vi "FF Target IN POLARIS Vision.vi"() -> ()   [LabVIEW 2009]
uses:
  IMAQdx Cam/IMAQdx Cam.lvclass
  XDisplay/POLARIS IMAQ Display.xctl
  XDisplay/Properties/ImageSource.ctl
  Utility/POLARIS Vision utility.lvlib
  Analyze Classes/Analyze Timer/Analyze Timer.lvclass
panel:
  in  "Amplifier":enum16{"CW", "A2", "A2 1.6x", "A3", "A4", "A5"}(ring)=enum."A4"
  out "error load settings":errorcluster
  in  "stop2":bool
  in  "Config Dir":path
  in  "Prefix":string
  in  "WorkDir":path
  out "XDisplay":cluster{"Image":T1}(xcontrol)
  in  "stop":bool
  in  "Camera Name":string
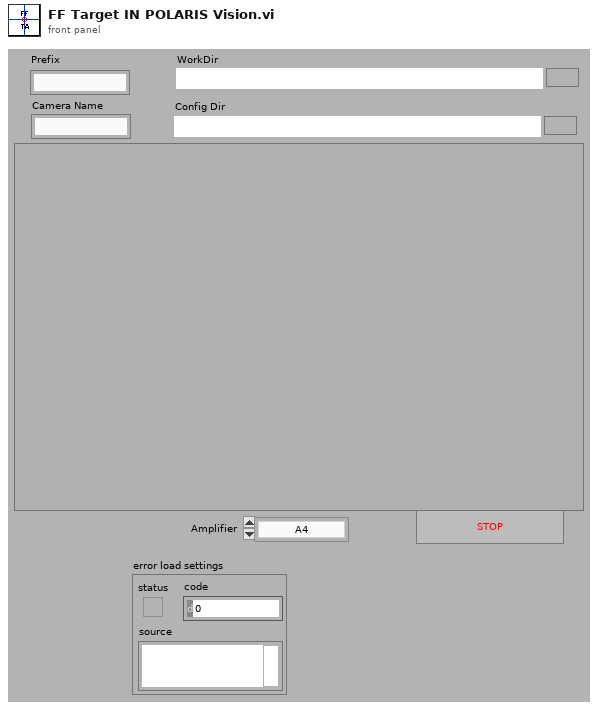
[diagram p1: front panel]
types:
  T1 = typedef "IMAQ Image.ctl" = refnum<image>
  T2 = typedef "POLARIS IMAQ Display.xctl/ImageSource.ctl" = enum16{"Camera", "File"}
  T3 = typedef "Image Type" = u32
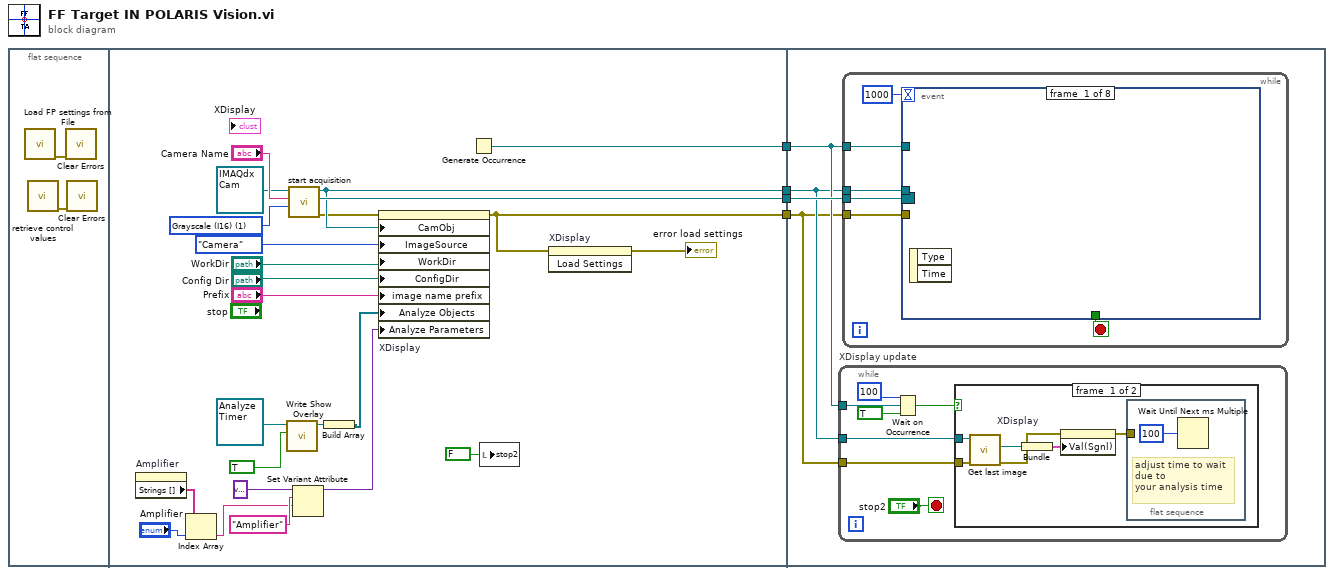
[diagram p0: block diagram]
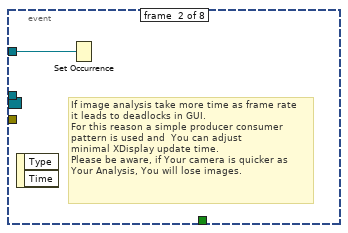
[diagram p3: hidden frame]
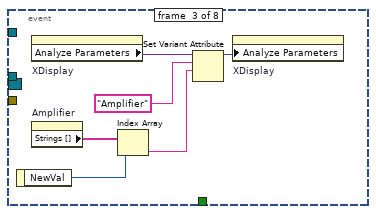
[diagram p4: hidden frame]
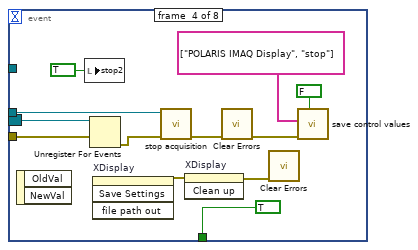
[diagram p5: hidden frame]
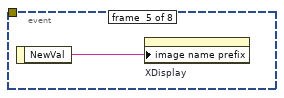
[diagram p6: hidden frame]
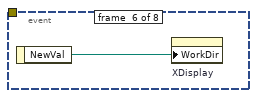
[diagram p7: hidden frame]
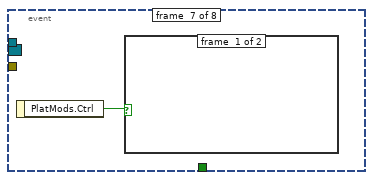
[diagram p8: hidden frame]
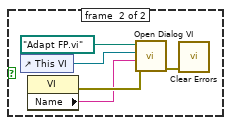
[diagram p9: hidden frame]
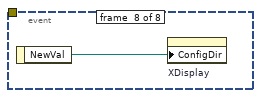
[diagram p10: hidden frame]
diagram:
  n1 = flat-sequence {
    tunnel: [w29] -> w4
    tunnel: [w25] -> w3
    tunnel: [w18] -> w2
    tunnel: [w20] -> w1
    tunnel: w4 -> [w34]
    tunnel: w3 -> [w32]
    tunnel: w2 -> [w31]
    tunnel: w1 -> [w33]
    frame #0 {
      n2 = call "Load FP settings from File.vi"() -> ("error out"=w5:errorcluster)  [unwired: 11 in]
      n3 = call "retrieve control values.vi"() -> ("error out"=w6:errorcluster)  [unwired: 10 in, 1 out]
      n4 = call <vilib>:"Clear Errors.vi"("error in (no error)"=w5) -> ()  [unwired: 6 in, 1 out]
      n5 = call <vilib>:"Clear Errors.vi"("error in (no error)"=w6) -> ()  [unwired: 6 in, 1 out]
    }
    frame #1 {
      w23 = T3 1 items=["Grayscale (U8)", "Grayscale (I16)", "Grayscale (SGL)", "Complex (CSG)", "RGB (U32)", "HSL (U32)", "RGB (U64)", "Grayscale (U16)"] ("Image Type")
      n6 = property on="Amplifier" class="Enum (strict)"() -> ("Strings []"=w8:string[])  [unwired: 2 in, 2 out]
      n7 = Index Array(array=w8, index="Amplifier") -> (element=w7:string)
      n8 = call-dynamic "Write Show Overlay.vi"("Overlay?"=TRUE, "Analyze BaseClass in"=refnum<class "Analyze Timer.lvclass"> refnum ("Analyze Timer.lvclass")) -> ("Analyze BaseClass out"=w15:refnum<class "Analyze Timer.lvclass">)  [unwired: 8 in, 1 out]
      n9 = call-dynamic "start acquisition.vi"("Image Type"=w23, "Camera Name"="Camera Name", "IMAQdx Cam in"=refnum<class "IMAQdx Cam.lvclass"> refnum ("IMAQdx Cam.lvclass")) -> ("error out"=w24:errorcluster, "Event Registration Refnum"=w29:refnum<event-registration>, "IMAQdx Cam out"=w25:refnum<class "IMAQdx Cam.lvclass">)  [unwired: 6 in]
      n10 = Set Variant Attribute(Variant=variant ("variant"), name="Amplifier", value=w7) -> (Variant out=w10:variant)  [unwired: 1 in, 2 out]
      n11 = Build Array(w15) -> (w14:refnum<class "Analyze Timer.lvclass">[])
      n12 = property on="XDisplay" class="POLARIS IMAQ Display (strict)"(error in=w24, "CamObj"=w25, "ImageSource"=ImageSource."Camera", "WorkDir"="WorkDir", "ConfigDir"="Config Dir", "image name prefix"="Prefix", "Analyze Objects"=w14, "Analyze Parameters"=w10) -> (error out=w18:errorcluster)  [unwired: 1 in, 1 out]
      n13 = Generate Occurrence() -> (w20:refnum<k4>)
      n14 = local write "stop2"(FALSE ("stop2")) -> ()
      n15 = invoke on="XDisplay" class="POLARIS IMAQ Display (strict)" method="Load Settings"(error in=w18) -> (error out=→"error load settings":errorcluster)  [unwired: 2 in, 2 out]
    }
    frame #2 {
      n16 = while "XDisplay update" {
        tunnel: w33 -> [w41]
        tunnel: w32 -> [w38]
        tunnel: w31 -> [w37]
        stop <- "stop2" stop-if-true
        n17 = Wait on Occurrence(1:TRUE ("ignore previous (T)"), 2:w41, 3:100 ("ms timeout (-1)")) -> (0:w39:bool)
        n18 = case shown="False" w39 {
          tunnel: w38 -> [w44 _]
          tunnel: w37 -> [w43 _]
          frame #0 {
            n19 = call-dynamic "Get last image.vi"("error in (no error)"=w43, "IMAQdx Cam in"=w44) -> ("error out"=w46:errorcluster, "Image Out"=w45:T1)  [unwired: 7 in, 1 out]
            n20 = Bundle("Image Out"=w45) -> (w47:cluster{"Image Out":T1})  [unwired: 1 in]
            n21 = property on="XDisplay" class="POLARIS IMAQ Display (strict)"(error in=w46, "Val(Sgnl)"=w47) -> (error out=w42:errorcluster)  [unwired: 1 in, 1 out]
            n22 = flat-sequence {
              tunnel: w42 -> [_]
              frame #0 {
                # "adjust time to wait\ndue to \nyour analysis time"
                n23 = Wait Until Next ms Multiple(millisecond multiple=u32 100 ("milliseconds to wait")) -> ()  [unwired: 1 out]
              }
            }
          }
          frame #1 {
          }
        }
      }
      n24 = while {
        tunnel: w32 -> [w53]
        tunnel: w34 -> [w52]
        tunnel: w31 -> [w51]
        tunnel: w33 -> [w50]
        stop <- w54 stop-if-true
        n25 = event shown="[6] \"Pane\": Mouse Down" {
          selector: w52 -> [_ _ _ w70 _ _ _ _]
          dyn-events: _ -> [_ _ _ _ _ _ _ _]
          timeout: 1000 -> [_ _ _ _ _ _ _ _]
          tunnel: [_ _ _ TRUE _ _ _ _] -> w54
          tunnel: w53 -> [_ _ _ w71 _ _ _ _]
          tunnel: w51 -> [_ _ _ w69 _ _ _ _]
          tunnel: w50 -> [_ w55 _ _ _ _ _ _]
          event #0 {
            n26 = event-data() -> ()  [unwired: 1 in, 2 out]
          }
          event #1 {
            # "If image analysis take more time as frame rate\nit leads to deadlocks in GUI.\nFor this reason a simple producer consumer \npattern is used and  You can adjust \nminimal XDisplay update time.\nPlease be aware, if Your camera is quicker as\nYour Analysis, You will lose images."
            n27 = event-data() -> ()  [unwired: 1 in, 2 out]
            n28 = Set Occurrence(w55) -> ()
          }
          event #2 {
            n29 = event-data() -> ("NewVal"=w60:enum16{"CW", "A2", "A2 1.6x", "A3", "A4", "A5"})  [unwired: 1 in]
            n30 = property on="XDisplay" class="POLARIS IMAQ Display (strict)"() -> ("Analyze Parameters"=w57:variant)  [unwired: 2 in, 2 out]
            n31 = property on="Amplifier" class="Enum (strict)"() -> ("Strings []"=w61:string[])  [unwired: 2 in, 2 out]
            n32 = Index Array(array=w61, index=w60) -> (element=w59:string)
            n33 = Set Variant Attribute(Variant=w57, name="Amplifier", value=w59) -> (Variant out=w56:variant)  [unwired: 1 in, 2 out]
            n34 = property on="XDisplay" class="POLARIS IMAQ Display (strict)"("Analyze Parameters"=w56) -> ()  [unwired: 2 in, 2 out]
          }
          event #3 {
            n35 = event-data() -> ()  [unwired: 1 in, 2 out]
            n36 = local write "stop2"(TRUE ("stop2")) -> ()
            n37 = Unregister For Events(event registration refnum=w70, error in=w69) -> (error out=w72:errorcluster)
            n38 = invoke on="XDisplay" class="POLARIS IMAQ Display (strict)" method="Save Settings"() -> (error out=w63:errorcluster)  [unwired: 4 in, 3 out]
            n39 = call-dynamic "stop acquisition.vi"("error in (no error)"=w72, "IMAQdx Cam in"=w71) -> ("error out"=w68:errorcluster)  [unwired: 8 in, 1 out]
            n40 = invoke on="XDisplay" class="POLARIS IMAQ Display (strict)" method="Clean up"(error in=w63) -> (error out=w62:errorcluster)  [unwired: 2 in, 2 out]
            n41 = call <vilib>:"Clear Errors.vi"("error in (no error)"=w68) -> ("error out"=w67:errorcluster)  [unwired: 6 in]
            n42 = call <vilib>:"Clear Errors.vi"("error in (no error)"=w62) -> ()  [unwired: 6 in, 1 out]
            n43 = call "save control values.vi"("Append timestamp (true)"=FALSE, "error in"=w67, "Dont save"=string[] ["POLARIS IMAQ Display", "stop"]) -> ()  [unwired: 5 in, 2 out]
          }
          event #4 {
            n44 = event-data() -> ("NewVal"=w74:string)  [unwired: 1 in]
            n45 = property on="XDisplay" class="POLARIS IMAQ Display (strict)"("image name prefix"=w74) -> ()  [unwired: 2 in, 2 out]
          }
          event #5 {
            n46 = event-data() -> ("NewVal"=w75:path)  [unwired: 1 in]
            n47 = property on="XDisplay" class="POLARIS IMAQ Display (strict)"("WorkDir"=w75) -> ()  [unwired: 2 in, 2 out]
          }
          event #6 {
            n48 = event-data() -> ("PlatMods.Ctrl"=w76:bool)  [unwired: 1 in]
            n49 = case shown="True" w76 {
              frame #0 {
              }
              frame #1 {
                n50 = control-ref of="This VI"() -> (w80:refnum<vi>)
                n51 = property class="VI"() -> (error out=w79:errorcluster, "Name"=w78:string)  [unwired: 2 in, 1 out]
                n52 = call "Open Dialog VI.vi"("error in"=w79, "Windows title"=w78, "ref for signalling"=w80, "vi path"=path "Adapt FP.vi") -> ("error out"=w77:errorcluster)  [unwired: 7 in]
                n53 = call <vilib>:"Clear Errors.vi"("error in (no error)"=w77) -> ()  [unwired: 6 in, 1 out]
              }
            }
          }
          event #7 {
            n54 = event-data() -> ("NewVal"=w82:path)  [unwired: 1 in]
            n55 = property on="XDisplay" class="POLARIS IMAQ Display (strict)"("ConfigDir"=w82) -> ()  [unwired: 2 in, 2 out]
          }
        }
      }
    }
  }
